vi "Get_Day_File_Client.vi"(4 "Use Hi Res Files":bool, 5 "Averaging Time (min)":dbl=5.0, 6 "End time":timestamp, 7 "Start time":timestamp, 8 "Channel Names":string[](array[string]), 9 "Data folder location":path=path "/G4-2-HD/Enflo Data/Server Day Files") -> (0 "Files with wrong times":path[](array[path]), 1 "All Channel Names":string[](array[string]), 2 "Data":dbl[][](array[numeric]), 3 "Times":dbl[](array[numeric]))   [LabVIEW 2015]
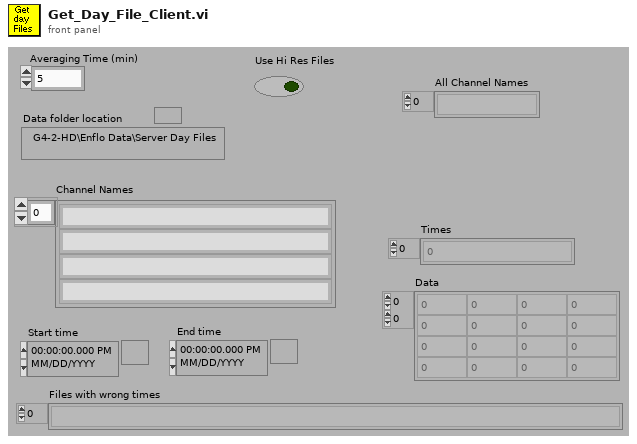
[diagram p1: front panel]
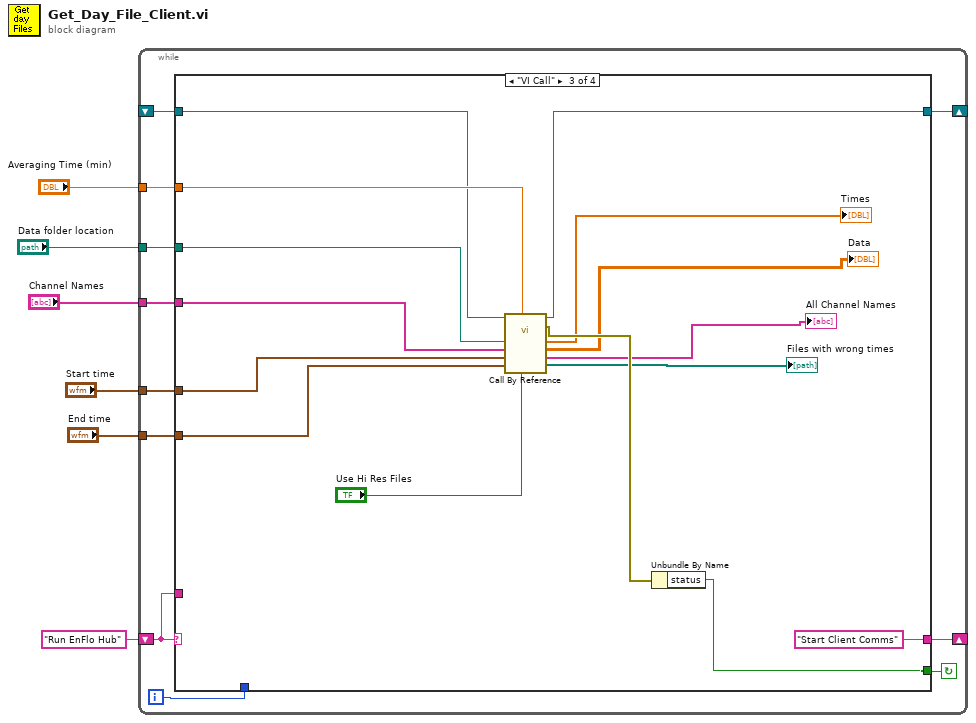
[diagram p0: block diagram]
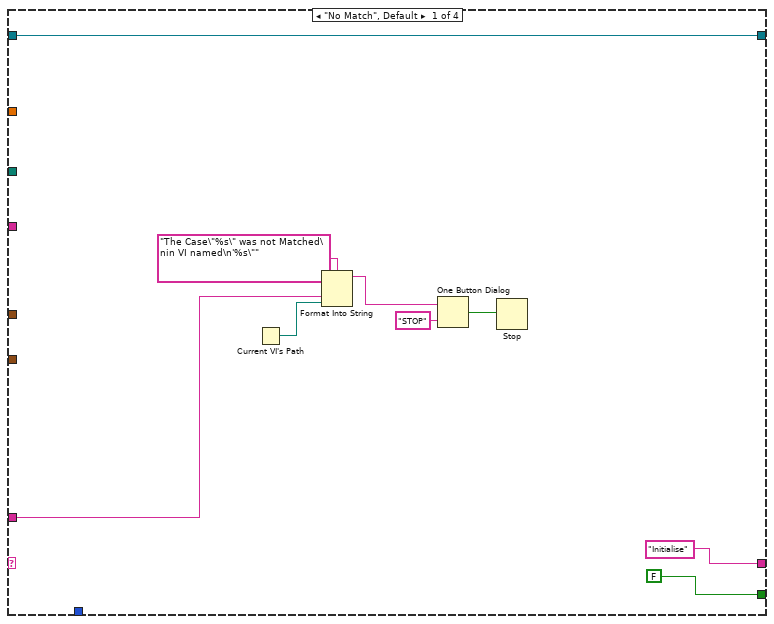
[diagram p2: hidden frame]
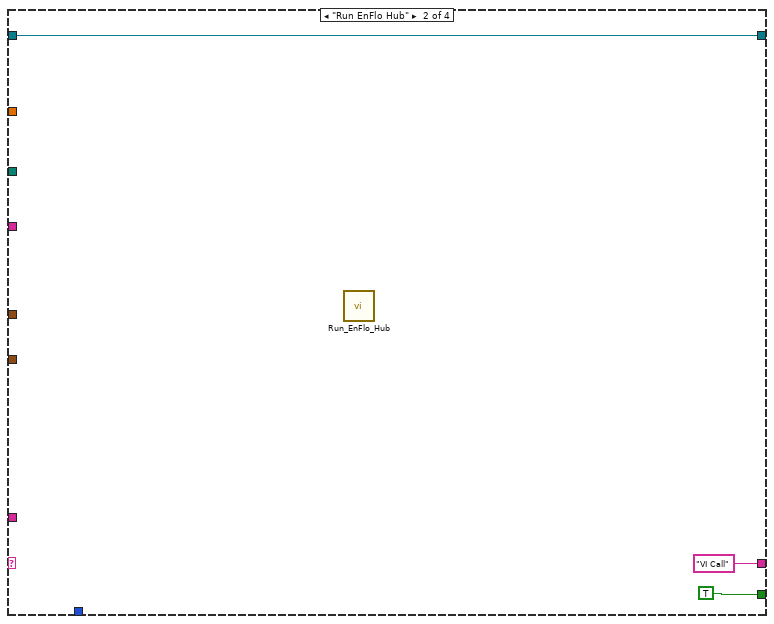
[diagram p3: hidden frame]
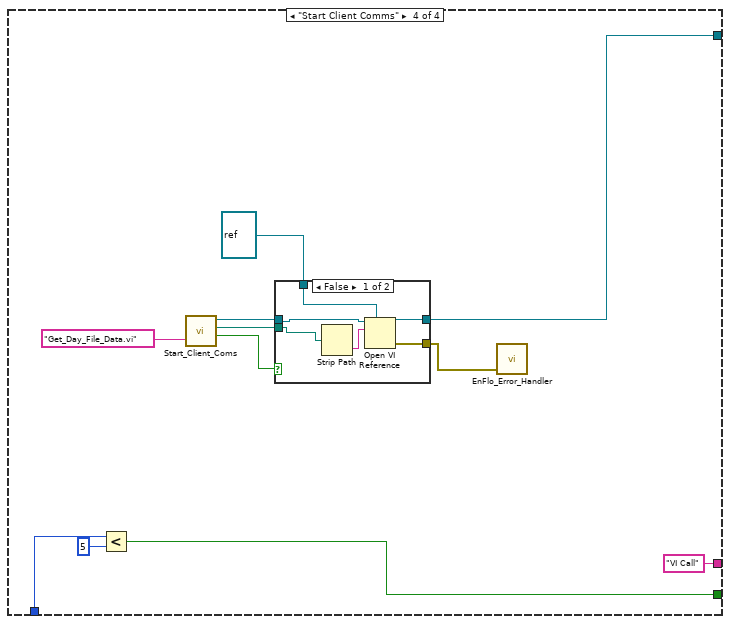
[diagram p4: hidden frame]
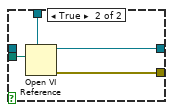
[diagram p5: hidden frame]
diagram:
  n1 = while {
    shift-left: "Run EnFlo Hub" -> [w15]
    shift-right: [w16] -> _
    shift-right: [w9] -> _
    shift-left: _ -> [w8]
    tunnel: "Data folder location" -> [w14]
    tunnel: "Channel Names" -> [w13]
    tunnel: "Start time" -> [w12]
    tunnel: "End time" -> [w11]
    tunnel: "Averaging Time (min)" -> [w10]
    i -> [w7]
    stop <- w17 continue-if-true
    n2 = case shown="\"VI Call\"" w15 {
      tunnel: [FALSE TRUE w37 w45] -> w17
      tunnel: ["Initialise" "VI Call" "Start Client Comms" "VI Call"] -> w16
      tunnel: w15 -> [w21 _ _ _]
      tunnel: w14 -> [_ _ w43 _]
      tunnel: w13 -> [_ _ w42 _]
      tunnel: w12 -> [_ _ w41 _]
      tunnel: w11 -> [_ _ w40 _]
      tunnel: w10 -> [_ _ w39 _]
      tunnel: [w18 w28 w31 w50] -> w9
      tunnel: w8 -> [w18 w28 w32 _]
      tunnel: w7 -> [_ _ _ w47]
      frame "No Match", Default {
        n3 = Current VI's Path() -> (path=w20:path)
        n4 = Format Into String(format string="The Case\"%s\" was not Matched\nin VI named\n'%s\"" ("Format String"), w21, w20) -> (resulting string=w24:string)  [unwired: 2 in, 1 out]
        n5 = One Button Dialog(message=w24, button name ("OK")="STOP") -> (true=w22:bool)
        n6 = Stop(stop? (T)=w22) -> ()
      }
      frame "Run EnFlo Hub" {
        n7 = call "Run_EnFlo_Hub.vi"() -> ()  [unwired: 8 out]
      }
      frame "VI Call" {
        n8 = call-by-ref "?"(reference=w32, "Use Hi Res Files"="Use Hi Res Files", "Averaging Time (min)"=w39, "End time"=w40, "Start time"=w41, "Channel Names"=w42, "Data folder location"=w43) -> (reference out=w31:refnum<vi>, error out=w38:errorcluster, "Files with wrong times"=→"Files with wrong times":path[], "All Channel Names"=→"All Channel Names":string[], "Data"=→"Data":dbl[][], "Times"=→"Times":dbl[])  [unwired: 1 in]
        n9 = Unbundle By Name(w38) -> ("status"=w37:bool)
      }
      frame "Start Client Comms" {
        n10 = Less?(x=w47, y=5) -> (x < y?=w45:bool)
        n11 = call "Start_Client_Coms.vi"("VI name to run on server"="Get_Day_File_Data.vi") -> ("LabVIEW application reference"=w53:refnum<vi>, "Checked VI name"=w55:path, "Local Call"=w54:bool)  [unwired: 1 in, 1 out]
        n12 = case shown="False" w54 {
          tunnel: refnum<vi> refnum ("trivial.vi type") -> [w57 w65]
          tunnel: w55 -> [w58 w64]
          tunnel: w53 -> [w56 _]
          tunnel: [w60 w63] -> w49
          tunnel: [w59 w62] -> w50
          frame False {
            n13 = Strip Path(path=w58) -> (name=w61:string)  [unwired: 1 out]
            n14 = Open VI Reference(type specifier VI Refnum (for type only)=w57, application reference (local)=w56, vi path=w61) -> (vi reference=w59:refnum<vi>, error out=w60:errorcluster)  [unwired: 1 in, 2 out]
          }
          frame True {
            n15 = Open VI Reference(type specifier VI Refnum (for type only)=w65, vi path=w64) -> (vi reference=w62:refnum<vi>, error out=w63:errorcluster)  [unwired: 1 in, 3 out]
          }
        }
        n16 = call "EnFlo_Error_Handler.vi"("error in (no error)"=w49) -> ()  [unwired: 2 in, 3 out]
      }
    }
  }
